vi "FPGA Test.vi"() -> ()   [LabVIEW 2025]
panel:
  out "Tick Count(Ticks)":u32
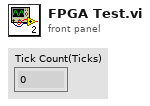
[diagram p1: front panel]
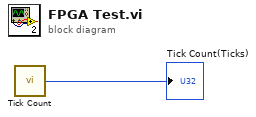
[diagram p0: block diagram]
diagram:
  n1 = call "Tick Count"() -> ("Tick Count(Ticks)"=→"Tick Count(Ticks)":u32)
